vi "Test Action Status.vi"(8 "error in (no error)":errorcluster, 11 "Instrument.Oxford1820 in":refnum<class "Instrument.Oxford1820.lvclass">) -> (0 "error out":errorcluster, 3 "Instrument.Oxford1820 out":refnum<class "Instrument.Oxford1820.lvclass">)   [LabVIEW 2019, in "Instrument.Oxford1820.lvclass"]
uses:
  Instrument.Oxford1820.lvclass
  <instrlib>/Mercury iXX/Public/Libraries/Magnet/Controls/PSU Actions.ctl
  Instrument.Oxford1820.lvclass/Instrument.Oxford1820.ctl
  <instrlib>/Mercury iXX/Public/Libraries/Magnet/Open/Open Magnet Device.vi
  <instrlib>/Mercury iXX/Public/Libraries/Magnet/Configuration/Read/PSU Action Status (Read).vi
  <instrlib>/Mercury iXX/Mercury iXX.lvlib
  <instrlib>/Mercury iXX/Public/Libraries/Magnet.lvlib
panel:
  out "PSU Act Stat":T1 caption="PSU Action Status"
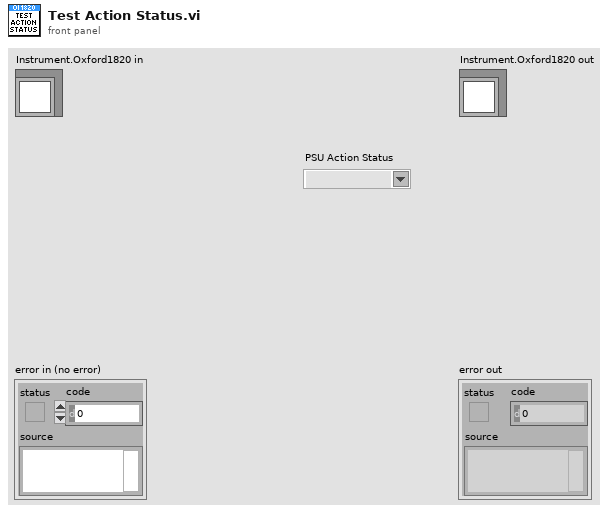
[diagram p1: front panel]
types:
  T1 = typedef "Mercury iXX.lvlib/Magnet.lvlib/PSU Actions.ctl" = string
  T2 = typedef "Mercury iXX.lvlib/Mercury Reference.ctl" = cluster{"Comms":refnum<visa-resource-name>, "Device ID":string[], "Comms Layer":T3, "Command":string, "Query reference":T4}
  T3 = typedef "Mercury iXX.lvlib/Comms Transport Layer.ctl" = enum16{"Ethernet TCP/IP", "USB", "ISOBus - RS-232", "GPIB"}
  T4 = typedef "Mercury iXX.lvlib/Query Dynamic Reference.ctl" = refnum<vi>
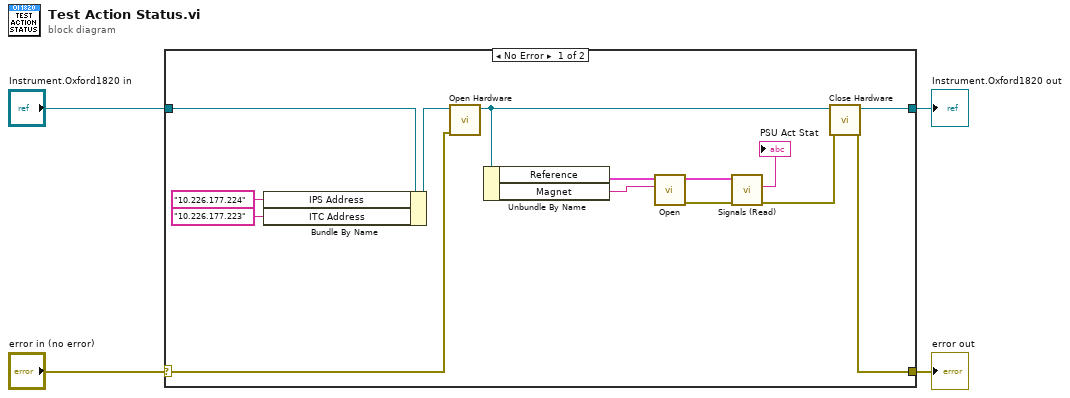
[diagram p0: block diagram]
diagram:
  n1 = case shown="No Error" "error in (no error)" {
    selector: "error in (no error)" -> [w17 w20]
    tunnel: [w5 w20] -> w3
    tunnel: [w18 w19] -> w1
    tunnel: "Instrument.Oxford1820 in" -> [w8 w19]
    frame No Error {
      n2 = Bundle By Name(cluster=w8, "IPS Address"="10.226.177.224" ("Configuration.IPS Address"), "ITC Address"="10.226.177.223" ("Configuration.ITC Address")) -> (w9:refnum<class "Instrument.Oxford1820.lvclass">)
      n3 = call-dynamic "Open Hardware.vi"("error in (no error)"=w17, "Instrument.Oxford1820 in"=w9) -> ("Instrument.Oxford1820 out"=w16:refnum<class "Instrument.Oxford1820.lvclass">)  [unwired: 8 in, 1 out]
      n4 = Unbundle By Name(w16) -> ("Reference"=w15:T2, "Magnet"=w14:string)
      n5 = call-poly <instrlib>:"Open.vi"("Device Identifier"=w14, "Mercury Reference In"=w15) -> ("error out"=w13:errorcluster, "Mercury Reference Out"=w6:T2)  [unwired: 8 in]
      n6 = call-poly <instrlib>:"Signals (Read).vi"("error in"=w13, "Mercury Reference In"=w6) -> ("error out"=w7:errorcluster, "PSU Act Stat"=→"PSU Act Stat":T1)  [unwired: 1 in, 7 out]
      n7 = call-dynamic "Close Hardware.vi"("error in (no error)"=w7, "Instrument.Oxford1820 in"=w16) -> ("error out"=w5:errorcluster, "Instrument.Oxford1820 out"=w18:refnum<class "Instrument.Oxford1820.lvclass">)  [unwired: 8 in]
    }
    frame Error {
    }
  }
  "error out" <- w3
  "Instrument.Oxford1820 out" <- w1
